vi "Main Loop.vi"(10 "AO in":refnum<class "Analog Output.lvclass">) -> ()   [LabVIEW 2017, in "Analog IO.lvlib" / "Analog Output.lvclass"]
uses:
  Analog Output.lvclass
  <vilib>/Platform/TimedLoop/XDataNode/timing_clust.ctl
  <vilib>/Platform/TimedLoop/XDataNode/nitl_modes.ctl
  <vilib>/Platform/TimedLoop/XDataNode/wakeup.ctl
  Analog Output.lvclass/Analog Output.ctl
  <vilib>/rvi/Emulation/niFpgaGetClockAttributes.vi
  <vilib>/rvi/Emulation/niFpgaSctlEmulationGetInTimedLoop.vi
  <vilib>/rvi/Emulation/niFpgaEmulationReportErrorSimple.vi
  <vilib>/rvi/DataTransferAndStorage/Container/Common/niFpgaContainerGetUniqueNameForEmu.vi
  <vilib>/rvi/DataTransferAndStorage/Container/Common/niFpgaContainerSetEmuInfo.vi
  <vilib>/rvi/eio/common/nirviEmuReportErrorAndStop.vi
  <vilib>/rvi/DataTransferAndStorage/Container/Common/niFpgaContainerExecOnDevCompGetState.vi
  <vilib>/rvi/Emulation/niFpgaEmulationIsFPGAContextNoSignature.vi
  <vilib>/rvi/Memory/Memory_Emulation/niFpgaMemoryEmulationCacheClearOnFirstRun.vi
  <vilib>/rvi/Memory/Memory_Emulation/nirvimemoryEmulationManagerCache_MakeExclusive.vi
  <vilib>/rvi/Memory/Memory_Emulation/niFpgaMemoryEmulationValidateCache.vi
  <vilib>/rvi/Memory/Memory_Emulation/nirvimemoryEmulationManagerCache_InsertValue.vi
  <vilib>/Utility/error.llb/Clear Errors.vi
  <vilib>/rvi/Memory/Memory_Emulation/nirvimemoryEmulationManagerCache_ReleaseExclusive.vi
  <vilib>/rvi/Memory/Memory_Emulation/nirvimemoryEmulationManagerCache_GetValue.vi
  <vilib>/rvi/Memory/Memory_Emulation/nirvimemoryEmulationManagerCache_SetValue.vi
  <vilib>/rvi/Emulation/niFpgaProcessEmulError.vi
  <vilib>/rvi/Emulation/niFpgaCriticalErrorInLSC.vi
  <vilib>/Platform/TimedLoop/XDataNode/XDataNode.xnode
  <vilib>/rvi/LocalResourceManager/LocalResourceManager.xnode
  <vilib>/rvi/DataTransferAndStorage/Container/XNode/niFpgaContainer.xnode
  <vilib>/rvi/DataTransferAndStorage/Register/Emulation/niFpgaRegisterEmulationRefIn.vi
  <vilib>/Platform/TimedLoop/XDataNode/XDNodeRunTimeDep.lvlib
  <instrlib>/_niInstr/Basic Elements/v1/FPGA/niInstr Basic Elements v1 FPGA.lvlib
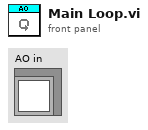
[diagram p1: front panel]
types:
  T1 = typedef "XDNodeRunTimeDep.lvlib/timing_clust.ctl" = cluster{"Expected End [f-1]":u64, "Actual End [f-1]":u64, "Finished Late? [f-1]":bool, "Expected End [i-1]":u64, "Actual End [i-1]":u64, "Finished Late? [i-1]":bool, "Expected Start [i]":u64, "Actual Start [i]":u64, "Expected Start [f]":u64, "Actual Start [f]":u64, "Source Name":string, "Structure Name":string, "Period":i64, "Deadline":i64, "Offset":i64, "Start":i64, "Priority":i32, "Timeout":i32, "Mode":T2, "Wakeup Reason":T3, "Error":errorcluster, "Source Type":string, "Secondary Source Type":string, "Global End Time":u64, "Global Start Time":u64, "Frame Duration":u64, "Iteration Duration":u64, "Assigned CPU":i32, "I/O Scan Engine Mode":u32}
  T2 = typedef "XDNodeRunTimeDep.lvlib/nitl_modes.ctl" = enum32{"No Change", "Process missed periods, maintain original phase", "Discard missed periods, maintain original phase", "Process missed periods, ignore original phase", "Discard missed periods, ignore original phase"}
  T3 = typedef "XDNodeRunTimeDep.lvlib/wakeup.ctl" = enum32{"Normal", "Aborted", "Asynchronous wakeup", "Timing source error", "Timed loop error", "Timeout"}
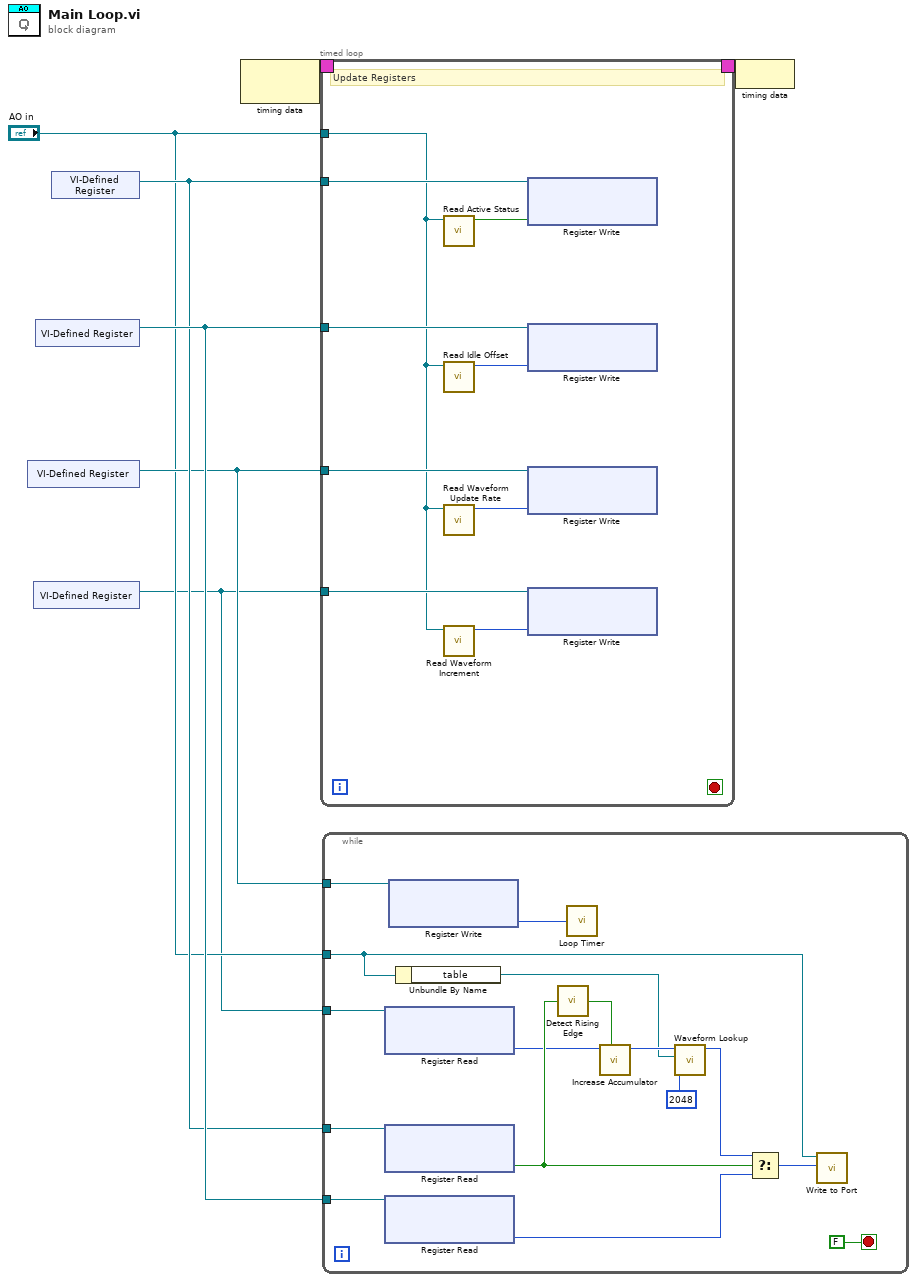
[diagram p0: block diagram]
diagram:
  n1 = xnode "VI-Defined Register"() -> ("Register Out"=w3:refnum<k21>)
  n2 = xnode "VI-Defined Register"() -> ("Register Out"=w1:refnum<k21>)
  n3 = xnode "VI-Defined Register"() -> ("Register Out"=w5:refnum<k21>)
  n4 = xnode "VI-Defined Register"() -> ("Register Out"=w4:refnum<k21>)
  n5 = node-c288() -> (w7:T1)  [unwired: 1 in]
  n6 = timed-loop {
    timing: w7 -> [_]
    timing-out: [_] -> w6
    tunnel: "AO in" -> [w8]
    tunnel: w5 -> [w16]
    tunnel: w4 -> [w14]
    tunnel: w3 -> [w11]
    tunnel: w1 -> [w10]
    stop <- _ stop-if-true
    # "Update Registers"
    n7 = call-dynamic "Read Active Status.vi"("AO in"=w8) -> ("active?"=w13:bool)  [unwired: 10 in]
    n8 = call-dynamic "Read Idle Offset.vi"("AO in"=w8) -> ("idle offset"=w15:i16)  [unwired: 10 in]
    n9 = call-dynamic "Read Waveform Update Rate.vi"("AO in"=w8) -> ("update rate"=w12:u32)  [unwired: 10 in]
    n10 = call-dynamic "Read Waveform Increment.vi"("AO in"=w8) -> ("increment"=w9:u32)  [unwired: 10 in]
    n11 = xnode ("Register Write")("Data"=w13, "Register In"=w14) -> ()  [unwired: 1 out]
    n12 = xnode ("Register Write")("Data"=w15, "Register In"=w16) -> ()  [unwired: 1 out]
    n13 = xnode ("Register Write")("Data"=w12, "Register In"=w11) -> ()  [unwired: 1 out]
    n14 = xnode ("Register Write")("Data"=w9, "Register In"=w10) -> ()  [unwired: 1 out]
  }
  n15 = while {
    tunnel: w5 -> [w33]
    tunnel: w4 -> [w32]
    tunnel: w3 -> [w30]
    tunnel: "AO in" -> [w20]
    tunnel: w1 -> [w23]
    stop <- FALSE stop-if-true
    n16 = xnode ("Register Read")("Register In"=w23) -> ("Data"=w22:u32)  [unwired: 1 out]
    n17 = xnode ("Register Read")("Register In"=w32) -> ("Data"=w26:bool)  [unwired: 1 out]
    n18 = xnode ("Register Read")("Register In"=w33) -> ("Data"=w31:i16)  [unwired: 1 out]
    n19 = xnode ("Register Write")("Register In"=w30) -> ("Data"=w29:u32)  [unwired: 1 out]
    n20 = Unbundle By Name(w20) -> ("table"=w24:refnum<k21>)
    n21 = call <instrlib>:"Detect Rising Edge.vi"("signal"=w26) -> ("edge detected"=w25:bool)  [unwired: 14 in]
    n22 = call "Loop Timer"("Count(Ticks)"=w29) -> ()  [unwired: 1 out]
    n23 = call "Increase Accumulator.vi"("reset"=w25, "increment"=w22) -> ("accumulator"=w27:u32)  [unwired: 9 in]
    n24 = call "Waveform Lookup.vi"("nelem"=u16 2048, "table"=w24, "accumulator"=w27) -> ("value"=w21:i16)  [unwired: 8 in]
    n25 = Select(t=w21, s=w26, f=w31) -> (s? t:f=w19:i16)
    n26 = call-dynamic "Write to Port.vi"("value"=w19, "AO in"=w20) -> ()  [unwired: 10 in]
  }
  n27 = node-c288(w6) -> ()
